vi "Mod_OFDM_Config_Pulse_Shaping.vi"(0 "Configuration in":variant, 7 "Pulse Shaping":T1={"System Filter"={"TX Filter"=enum."Raised Cosine", "Alpha"=0.5, "filter length"=8}, "Modulation system parameters"={"samples per symbol (16)"=16}, "symbol rate (Hz)"=100000.0} {"symbol rate (Hz)" min=1.0 step=1.0 format="%.2p"; "Modulation system parameters"."samples per symbol (16)" step=2; "System Filter"."Alpha" min=0.0 max=1.0 step=0.05 format="%.2f"}, 11 "error in":errorcluster) -> (4 "Configuration out":variant, 8 "Pulse Shaping":T1={"System Filter"={"TX Filter"=enum."Raised Cosine", "Alpha"=0.5, "filter length"=8}, "Modulation system parameters"={"samples per symbol (16)"=16}, "symbol rate (Hz)"=100.0} {"symbol rate (Hz)" min=1.0 step=1.0 format="%.2p"; "Modulation system parameters"."samples per symbol (16)" step=2; "System Filter"."Alpha" min=0.0 max=1.0 step=0.05 format="%.2f"}, 15 "error out":errorcluster)   [LabVIEW 2010]
uses:
  Controls(Type_DEf)/Configure Pulse Shaping.ctl
panel:
  out "Filter Coefficients":dbl[](graph)
  in  "Cancel Operation":bool
  in  "Apply Settings":bool
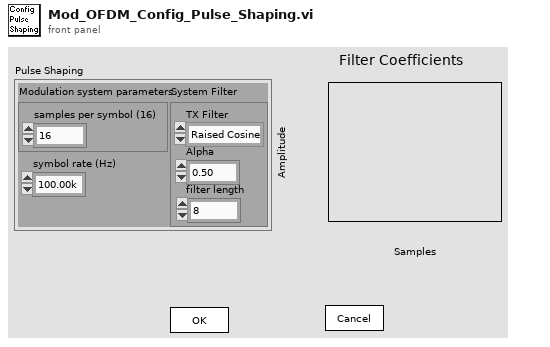
[diagram p1: front panel]
types:
  T1 = typedef "Configure Pulse Shaping.ctl" = cluster{"System Filter":cluster{"TX Filter":enum16{"none", "Raised Cosine", "Root Raised Cos"}, "Alpha":dbl, "filter length":i32}, "Modulation system parameters":cluster{"samples per symbol (16)":u32}, "symbol rate (Hz)":dbl}
  T2 = cluster{"System Filter":cluster{"TX Filter":enum16{"none", "Raised Cosine", "Root Raised Cos"}, "Alpha":dbl, "filter length":i32}, "Modulation system parameters":cluster{"samples per symbol (16)":u32}, "symbol rate (Hz)":dbl}
  T3 = enum16{"none", "Raised Cosine", "Root Raised Cos"}
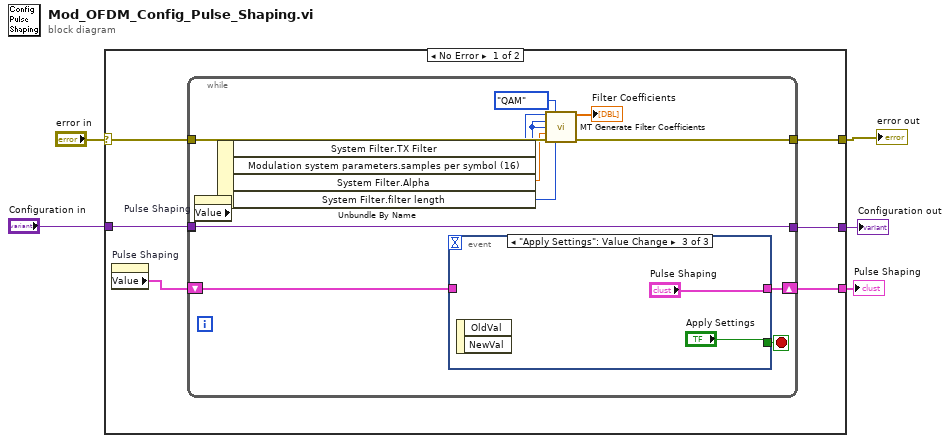
[diagram p0: block diagram]
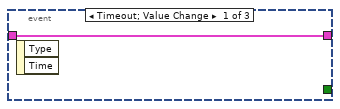
[diagram p2: hidden frame]
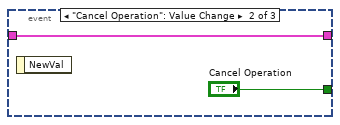
[diagram p3: hidden frame]
diagram:
  n1 = case shown="No Error" "error in" {
    selector: "error in" -> [w7 w30]
    tunnel: [w11 _] -> w5
    tunnel: [w10 w30] -> w4
    tunnel: "Configuration in" -> [w9 _]
    tunnel: [w8 _] -> w2
    frame No Error {
      n2 = property on="Pulse Shaping" class="Clust (strict)"() -> ("Value"=w6:T2)  [unwired: 2 in, 2 out]
      n3 = while {
        shift-right: [w24] -> w11
        shift-left: w6 -> [w21]
        tunnel: w7 -> [w20]
        tunnel: [w19] -> w10
        tunnel: [w22] -> _
        tunnel: w9 -> [w22]
        tunnel: [w22] -> w8
        stop <- w23 stop-if-true
        n4 = property on="Pulse Shaping" class="Clust (strict)"() -> ("Value"=w13:T2)  [unwired: 2 in, 2 out]
        n5 = Unbundle By Name(w13) -> ("System Filter.TX Filter"=w18:T3, "Modulation system parameters.samples per symbol (16)"=w17:u32, "System Filter.Alpha"=w16:dbl, "System Filter.filter length"=w15:i32)
        n6 = event shown="[2] \"Apply Settings\": Value Change" {
          selector: _ -> [_ _ _]
          dyn-events: _ -> [_ _ _]
          timeout: _ -> [_ _ _]
          tunnel: [w25 w26 "Pulse Shaping"] -> w24
          tunnel: w21 -> [w25 w26 _]
          tunnel: [_ "Cancel Operation" "Apply Settings"] -> w23
          event Timeout; Value Change {
            n7 = event-data() -> ()  [unwired: 1 in, 2 out]
          }
          event "Cancel Operation": Value Change {
            n8 = event-data() -> ()  [unwired: 1 in, 1 out]
          }
          event "Apply Settings": Value Change {
            n9 = event-data() -> ()  [unwired: 1 in, 2 out]
          }
        }
        n10 = call <vilib>:"MT Generate Filter Coefficients.vi"("pulse shaping filter (none)"=w18, "modulation type"=enum16{"FSK", "PSK", "QAM", "MSK", "PAM", "ASK"}."QAM", "pulse shaping samples per symbol (16)"=w17, "matched samples per symbol (16)"=w17, "filter parameter"=w16, "error in (no error)"=w20, "filter length (symbols)"=w15) -> ("pulse shaping filter coefficients"=→"Filter Coefficients":dbl[], "error out"=w19:errorcluster)  [unwired: 6 in, 1 out]
      }
    }
    frame Error {
    }
  }
  "error out" <- w4
  "Pulse Shaping" <- w5
  "Configuration out" <- w2
